vi "Pre Launch Init.vi"(11 "ClientUI in":refnum<class "ClientUI.lvclass">) -> (0 "error out":errorcluster, 3 "ClientUI out":refnum<class "ClientUI.lvclass">)   [LabVIEW 2018, in "ClientUI.lvlib" / "ClientUI.lvclass"]
doc: "(<B>Filename</B>: Actor Framework.lvlib:Actor.lvclass:Pre Launch Init.vi)\n\nDefines behavior that occurs after the Launch Nested Actor method is invoked but before the actor's Actor Core method begins running.\n\nBy default, this method does nothing. A descendant class may override it to define behavior."
uses:
  ClientUI.lvclass
  C:/Program Files/National Instruments/LabVIEW 2018/vi.lib/ActorFramework/Actor/Actor.lvclass
  TCP_Client/TCP_Client Messages/Read Msg/Read Msg.lvclass
  C:/Program Files/National Instruments/LabVIEW 2018/vi.lib/ActorFramework/Message/Message.lvclass
  <vilib>/ActorFramework/Actor/Actor.lvclass/Actor.ctl
  <vilib>/ActorFramework/Message Enqueuer/Message Enqueuer.lvclass/Message Enqueuer.ctl
  ClientUI.lvclass/ClientUI.ctl
  <vilib>/ActorFramework/Message Enqueuer/Init from Existing Queue.vi
  TCP_Client/TCP_Client/TCP_Client.lvclass
  <vilib>/ActorFramework/Message Enqueuer/Message Enqueuer.lvclass
  <vilib>/ActorFramework/Actor/Actor.lvclass
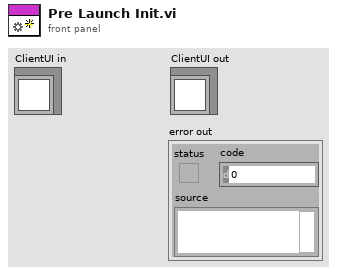
[diagram p1: front panel]
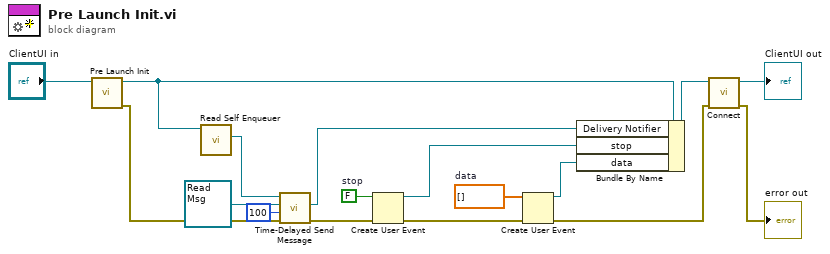
[diagram p0: block diagram]
diagram:
  w14 = dbl[] []  # data
  w15 = FALSE  # stop
  n1 = call-parent "Pre Launch Init.vi"("Actor in"="ClientUI in") -> ("error out"=w9:errorcluster, "Actor out"=w8:refnum<class "ClientUI.lvclass">)  [unwired: 9 in]
  n2 = call <vilib>:"Read Self Enqueuer.vi"("Actor"=w8) -> ("Self Enqueuer"=w7:refnum<class "Message Enqueuer.lvclass">)  [unwired: 10 in]
  n3 = call <vilib>:"Time-Delayed Send Message.vi"("error in (no error)"=w9, "Milliseconds To Wait"=100, "Message"=refnum<class "Read Msg.lvclass"> refnum ("TCP_Client.lvlib:Read Msg.lvclass"), "Message Enqueuer"=w7) -> ("error out"=w10:errorcluster, "Delivery Notifier"=w5:refnum<notifier>)  [unwired: 6 in]
  n4 = Create User Event(user event datatype=w15, error in=w10) -> (user event=w13:refnum<user-event>, error out=w16:errorcluster)
  n5 = Create User Event(user event datatype=w14, error in=w16) -> (user event=w12:refnum<user-event>, error out=w2:errorcluster)
  n6 = Bundle By Name(cluster=w8, "Delivery Notifier"=w5, "stop"=w13, "data"=w12) -> (w3:refnum<class "ClientUI.lvclass">)
  n7 = call-dynamic "Connect.vi"("error in (no error)"=w2, "TCP_Client in"=w3) -> ("error out"=→"error out":errorcluster, "TCP_Client out"=→"ClientUI out":refnum<class "ClientUI.lvclass">)  [unwired: 8 in]
